vi "Do.vi"(8 "error in (no error)":errorcluster, 10 "Actor in":refnum<class "Actor.lvclass">, 11 "UpdateIsOverRange Msg":refnum<class "UpdateIsOverRange Msg.lvclass">) -> (0 "error out":errorcluster, 2 "Actor out":refnum<class "Actor.lvclass">)   [LabVIEW 2013, in "CS++DMMGui.lvlib" / "UpdateIsOverRange Msg.lvclass"]
doc: "(<B>Filename</B>: Actor Framework.lvlib:Message.lvclass:Do.vi)\n\nDefines what a message does when it is received by an actor. Generally, a message instructs an actor to invoke one of its methods.\n\nBy default, this method does nothing. A child class must override it to define behavior. Create a child class by using the Actor Framework Message Maker dialog box."
uses:
  UpdateIsOverRange Msg.lvclass
  <vilib>/ActorFramework/Actor/Actor.lvclass
  CS++DMMGui/CS++DMMGui.lvclass
  Core/Actors/CS++PVMonitor Messages/CS++PVUpdate Msg/CS++PVUpdate Msg.lvclass/CS++PVUpdate Msg.ctl
  Core/Classes/CS++ProcessVariables/ProcessVariable/PV.lvclass/PV.ctl
  Core/Classes/CS++ProcessVariables/ProcessVariable/PV.lvclass
  Core/Actors/CS++PVMonitor Messages/CS++PVUpdate Msg/CS++PVUpdate Msg.lvclass
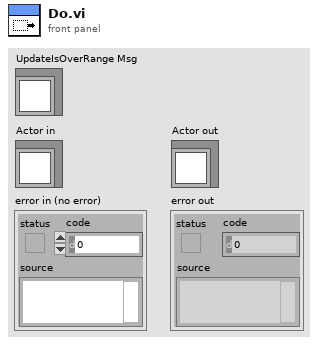
[diagram p1: front panel]
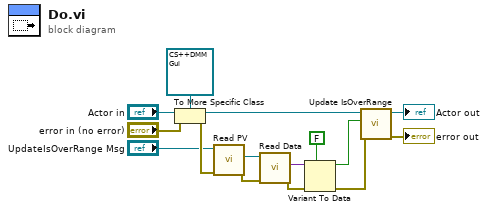
[diagram p0: block diagram]
diagram:
  n1 = To More Specific Class(target class=refnum<class "CS++DMMGui.lvclass"> refnum ("CS++DMMGui.lvlib:CS++DMMGui.lvclass"), reference="Actor in", error in="error in (no error)") -> (specific class reference=w5:refnum<class "CS++DMMGui.lvclass">, error out=w11:errorcluster)
  n2 = call "Read PV.vi"("error in (no error)"=w11, "CS++PVUpdate Msg in"="UpdateIsOverRange Msg") -> ("error out"=w14:errorcluster, "PV"=w15:refnum<class "PV.lvclass">)  [unwired: 7 in, 1 out]
  n3 = call "Read Data.vi"("error in (no error)"=w14, "PV in"=w15) -> ("error out"=w13:errorcluster, "Data"=w12:variant)  [unwired: 7 in, 1 out]
  n4 = Variant To Data(error in=w13, type=FALSE, Variant=w12) -> (data=w3:bool, error out=w4:errorcluster)
  n5 = call "Update IsOverRange.vi"("error in (no error)"=w4, "is over-range"=w3, "CS++DMMGui in"=w5) -> ("error out"=→"error out":errorcluster, "CS++DMMGui out"=→"Actor out":refnum<class "CS++DMMGui.lvclass">)  [unwired: 7 in]
